vi "Translate_Coordinate.vi"(0 "Input Data":dbl[](array[numeric])) -> (1 "Translation Matrix":T1, 2 "Translated Data":dbl[](array[numeric]))   [LabVIEW 2011]
uses:
  <vilib>/Analysis/Matrix/Datatypes/RealMatrix.ctl
  <vilib>/Analysis/baseanly.llb/A x Vector.vi
  <vilib>/Analysis/NI_AALBase.lvlib
  <vilib>/Analysis/Matrix/NI_Matrix.lvlib
panel:
  # "X"
  # "="
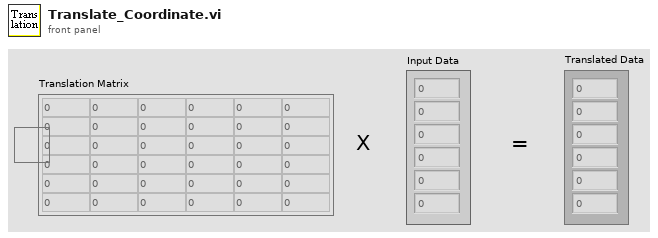
[diagram p1: front panel]
types:
  T1 = typedef "NI_Matrix.lvlib/RealMatrix.ctl" = dbl[][]
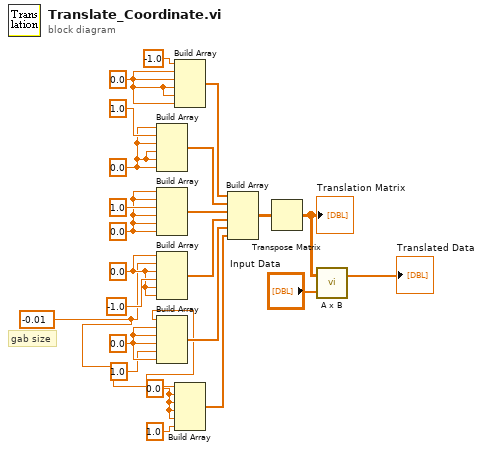
[diagram p0: block diagram]
diagram:
  w1 = -0.01 ("원소")
  w14 = 0.0 ("원소")
  w15 = 0.0 ("원소")
  w18 = 0.0 ("원소")
  w19 = 0.0 ("원소")
  w2 = 0.0 ("원소")
  w3 = 0.0 ("원소")
  # "gab size"
  n1 = Build Array(w2, 1.0 ("원소"), w2, w2, w2, w2) -> (w11:dbl[])
  n2 = Build Array(w19, w19, 1.0 ("원소"), w19, w19, w19) -> (w10:dbl[])
  n3 = Build Array(w15, w1, w15, -1.0 ("원소"), w15, w15) -> (w9:dbl[])
  n4 = Build Array(w1, w14, w14, w14, 1.0 ("원소"), w14) -> (w8:dbl[])
  n5 = Build Array(-1.0 ("원소"), w3, w3, w3, w3, w3) -> (w12:dbl[])
  n6 = Build Array(w18, w18, w18, w18, w18, 1.0 ("원소")) -> (w7:dbl[])
  n7 = Build Array(w12, w11, w10, w9, w8, w7) -> (w23:T1)
  n8 = Transpose Matrix(1:w23) -> (0:w6:T1)
  "Translation Matrix" <- w6
  n9 = call-poly <vilib>:"A x B.vi"("Vector"="Input Data", "A"=w6) -> ("A x Vector"=→"Translated Data":dbl[])  [unwired: 1 out]
